vi "Update Progress Bar.vi"(7 "Action":T1=enum."Set to Value", 8 "error in (no error)":errorcluster, 10 "Value":u8) -> (0 "error out":errorcluster)   [LabVIEW 2013, in "Progress Bar.lvlib"]
uses:
  Progress Bar.lvlib
  Controls/Update Bar Actions.ctl
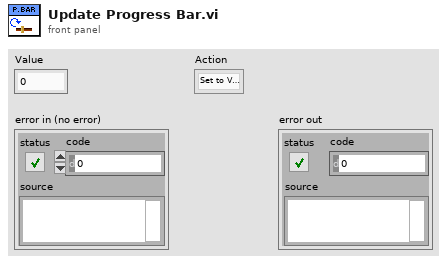
[diagram p1: front panel]
types:
  T1 = typedef "Progress Bar.lvlib/Update Bar Actions.ctl" = enum16{"Add To Existing", "Set to Value"}
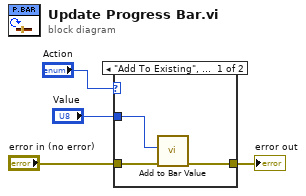
[diagram p0: block diagram]
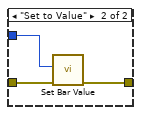
[diagram p2: hidden frame]
diagram:
  n1 = case shown="\"Add To Existing\", Default" "Action" {
    tunnel: "Value" -> [w7 w10]
    tunnel: "error in (no error)" -> [w6 w9]
    tunnel: [w5 w8] -> w1
    frame "Add To Existing", Default {
      n2 = call "Add to Bar Value.vi"("error in (no error)"=w6, "Amount to Add"=w7) -> ("error out"=w5:errorcluster)  [unwired: 9 in]
    }
    frame "Set to Value" {
      n3 = call "Set Bar Value.vi"("error in (no error)"=w9, "Slider Value"=w10) -> ("error out"=w8:errorcluster)  [unwired: 9 in]
    }
  }
  "error out" <- w1
